vi "Main.vi"(8 "MaxPulse_Path":path, 9 "SingleMeasurement_Path":path, 10 "Optometer cfg file":path=path "C:/Gigahertz-Optik/config/TR9600MPEconfig.gdf", 11 "deviceName":string="TR9600_57976") -> (0 "Pulse End (ms)":dbl format="%.4f", 1 "Pulse Begin (ms)":dbl format="%.4f", 2 "Pulse_Time (µs)":dbl format="%.2f", 3 "Pulse_Energy (V/s)":dbl)   [LabVIEW 2018]
uses:
  <userlib>/Gigahertz-Optik/GOMDTR9600/GOMDTR9600.lvlib
panel:
  out "Progress":i32
  out "Single Measurement":cluster{dbl[], dbl[]}(graph) caption="Spectrum"
  out "State":i32
  in  "Resolution":u32=10000000
  out "Maximum Pulse":cluster{i32[], dbl[]}(graph) caption="Spectrum"
  out "Status":string
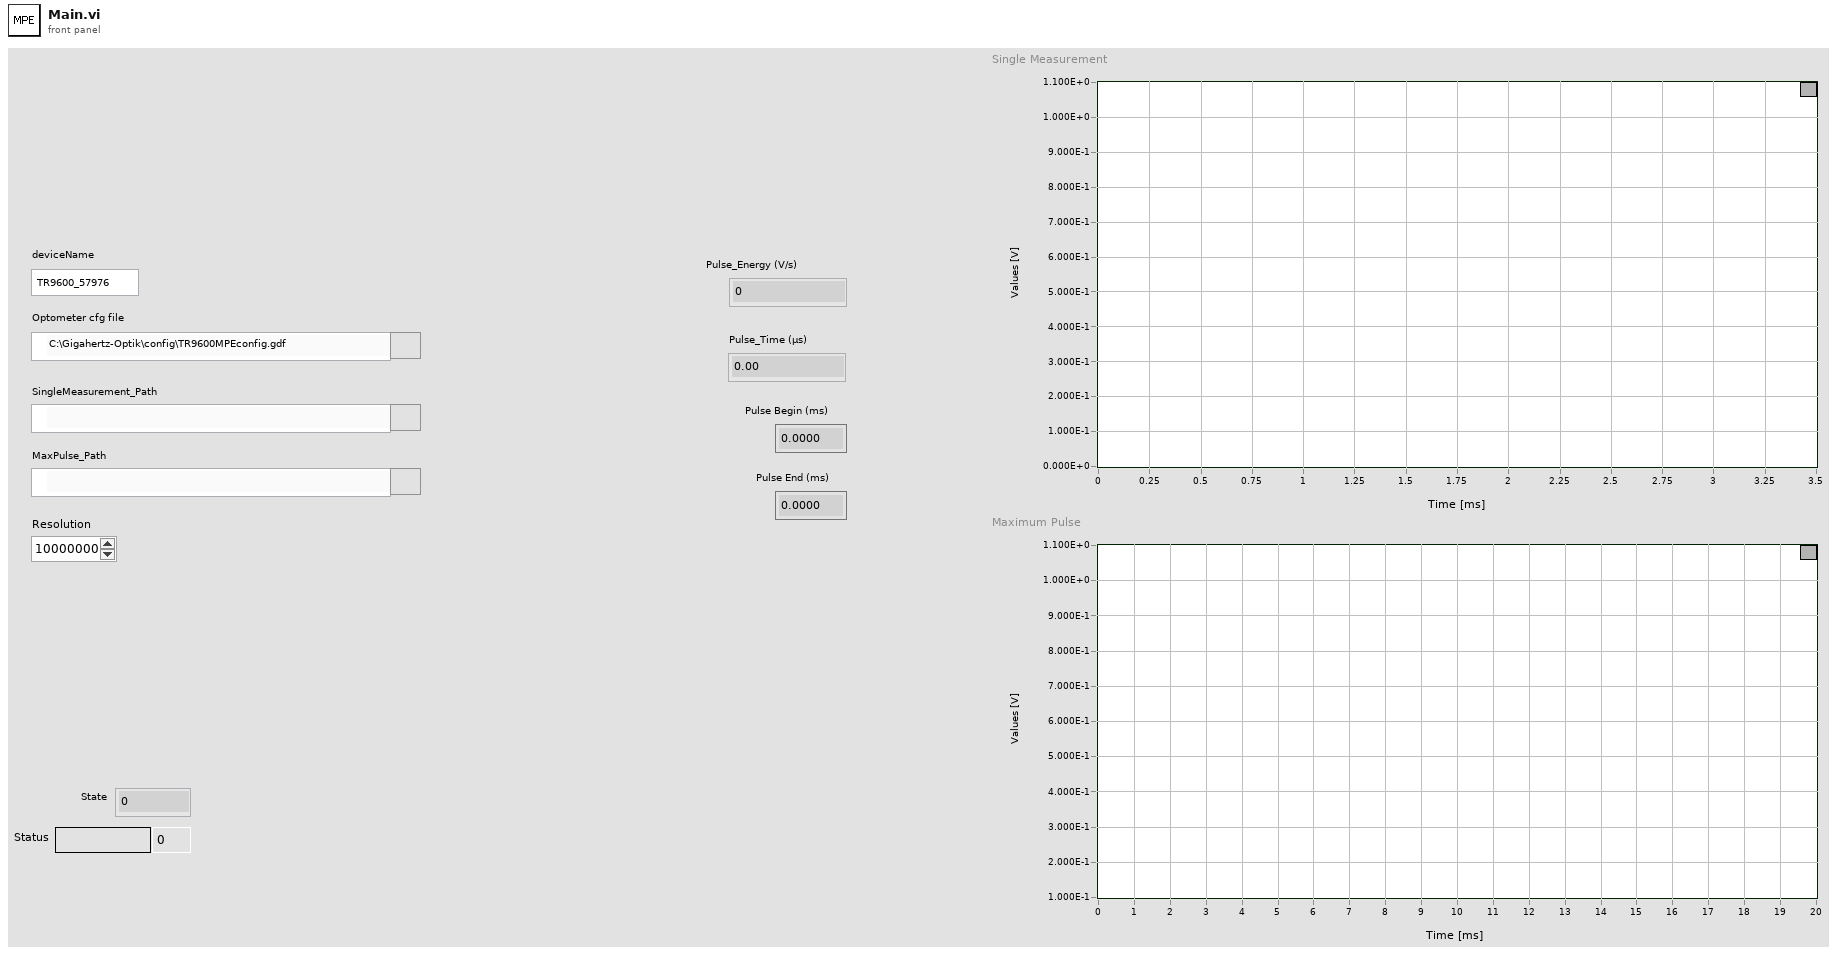
[diagram p1: front panel]
types:
  T1 = cluster{"address":i32, "mean value":dbl, "min value":dbl, "max value":dbl}[][]
  T2 = typedef "imagedata.ctl" = cluster{"image type":i32, "image depth":i32, "image":u8[], "mask":u8[], "colors":u32[], "Rectangle":cluster{"left":i16, "top":i16, "right":i16, "bottom":i16}}
  T3 = enum32{"invalid app kind", "Development System", "Run Time System", "Student Edition", "Embedded LabVIEW", "Evaluation", "Custom"}
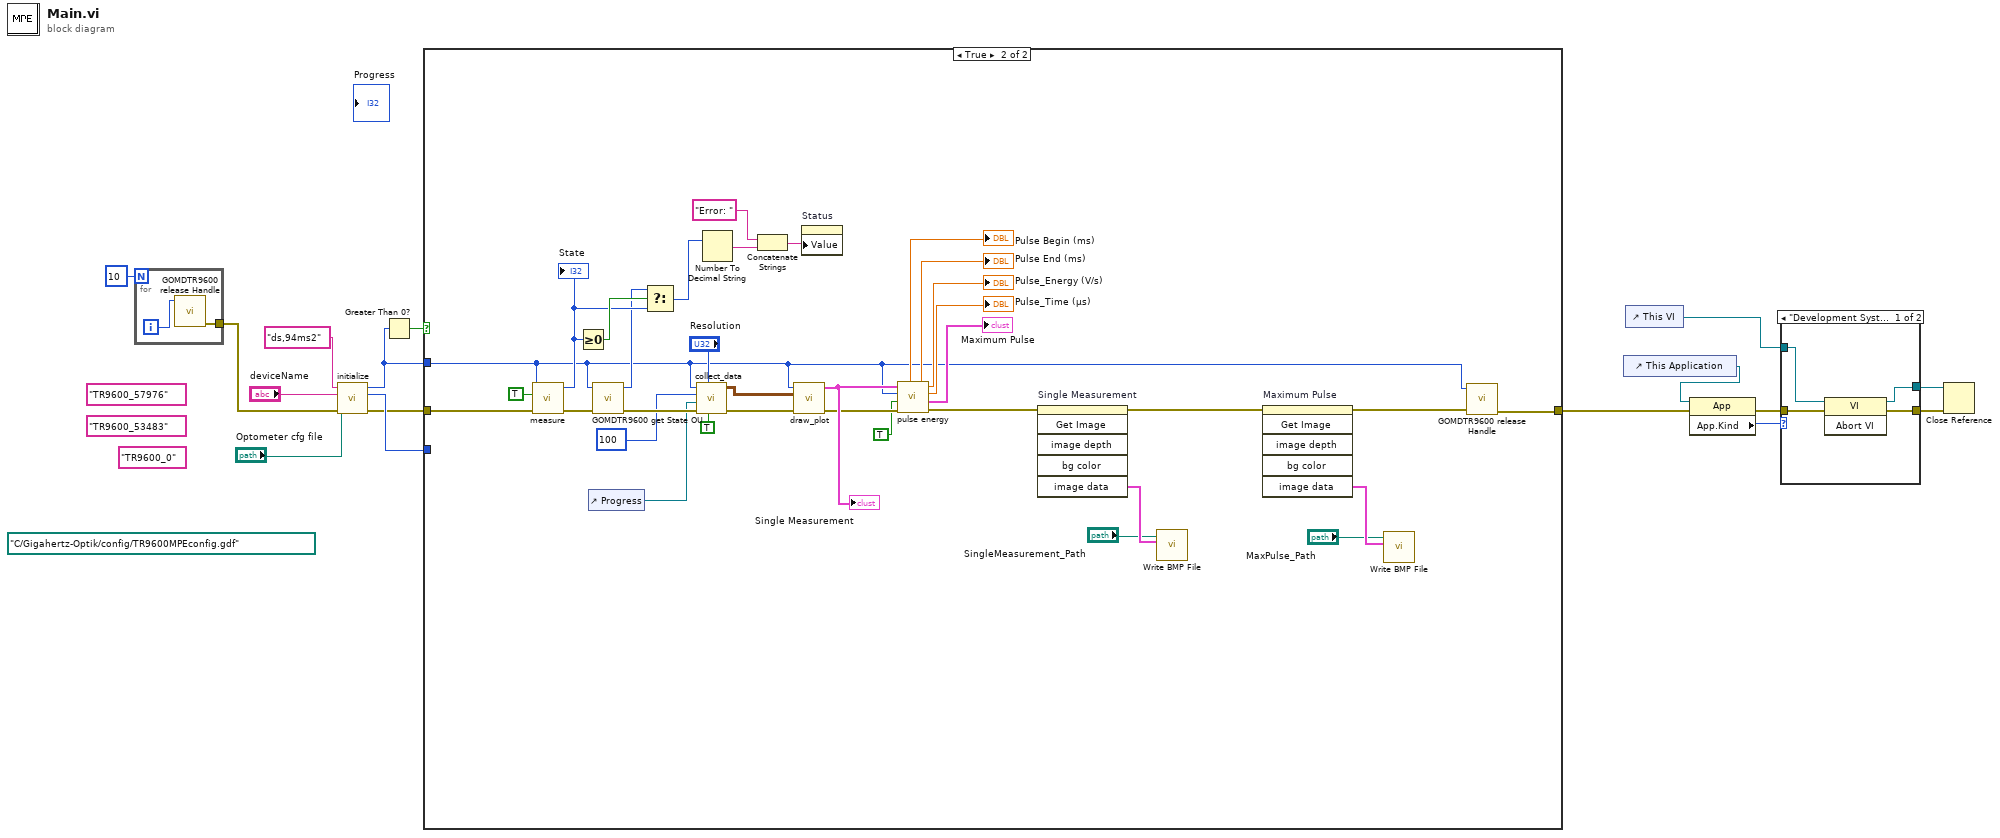
[diagram p0: block diagram]
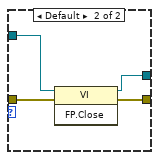
[diagram p2: hidden frame]
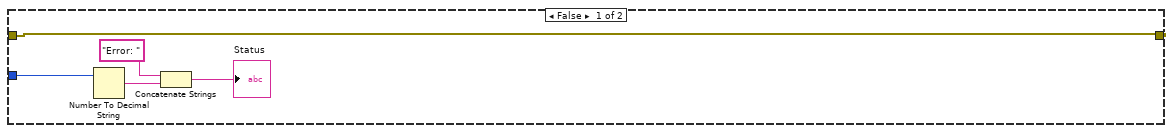
[diagram p3: hidden frame]
diagram:
  (unwired) "TR9600_53483" ("deviceName")
  (unwired) "TR9600_57976" ("deviceName")
  (unwired) path "C:/Gigahertz-Optik/config/TR9600MPEconfig.gdf" ("filename")
  (unwired) "TR9600_0" ("deviceName")
  n1 = for {
    N: 10 -> [_]
    tunnel: [w17] -> w4
    i -> [w18]
    n2 = call <userlib>:"GOMDTR9600 release Handle.vi"("handle"=w18) -> ("error out"=w17:errorcluster)  [unwired: 9 in, 1 out]
  }
  n3 = call "initialize.vi"("error in (no error)"=w4, "Optometer cfg file"="Optometer cfg file", "deviceName"="deviceName", "password"="ds,94ms2") -> ("error out"=w6:errorcluster, "function return"=w7:i32, "handle"=w3:i32)  [unwired: 5 in]
  n4 = Greater Than 0?(x=w3) -> (x > 0?=w16:bool)
  n5 = case shown="True" w16 {
    tunnel: w3 -> [_ w31]
    tunnel: w6 -> [w19 w57]
    tunnel: w7 -> [w23 _]
    tunnel: [w19 w32] -> w10
    frame False {
      n6 = Number To Decimal String(number=w23) -> (decimal integer string=w21:string)  [unwired: 1 in]
      n7 = Concatenate Strings("Error: ", w21) -> (→"Status":string)
    }
    frame True {
      n8 = call "measure.vi"("error in (no error)"=w57, "Measure"=TRUE, "handle"=w31) -> ("error out"=w52:errorcluster, "state"=w49:i32)  [unwired: 7 in]
      "State" <- w49
      n9 = Greater Or Equal To 0?(x=w49) -> (x >= 0?=w50:bool)
      n10 = control-ref of="Progress"() -> (w46:refnum<vi>)
      n11 = call <userlib>:"GOMDTR9600 get State OU.vi"("error in (no error)"=w52, "handle"=w31) -> ("error out"=w51:errorcluster, "value"=w48:i32)  [unwired: 7 in, 1 out]
      n12 = Select(t=w48, s=w50, f=w49) -> (s? t:f=w47:i32)
      n13 = call "collect_data.vi"("data?"=TRUE, "Resolution"="Resolution", "error in (no error)"=w51, "progress"=w46, "No. of values"=100, "handle"=w31) -> ("error out"=w56:errorcluster, "Dataset"=w42:T1)  [unwired: 4 in]
      n14 = Number To Decimal String(number=w47) -> (decimal integer string=w53:string)  [unwired: 1 in]
      n15 = Concatenate Strings("Error: ", w53) -> (w55:string)
      n16 = call "draw_plot.vi"("error in (no error)"=w56, "Dataset"=w42, "handle"=w31) -> ("error out"=w37:errorcluster, "Plot"=w38:cluster{dbl[], dbl[]})  [unwired: 7 in]
      "Single Measurement" <- w38
      n17 = property on="Status" class="Str"("Value"=w55) -> ()  [unwired: 2 in, 2 out]
      n18 = call "pulse energy.vi"("error in (no error)"=w37, "Boolean"=TRUE, "handle"=w31, "Spectrum"=w38) -> ("error out"=w26:errorcluster, "MaxPulse"=→"Maximum Pulse":cluster{i32[], dbl[]}, "Pulse_time"=→"Pulse_Time (µs)":dbl, "PulseEnergy"=→"Pulse_Energy (V/s)":dbl, "Pulse End"=→"Pulse End (ms)":dbl, "Pulse Begin"=→"Pulse Begin (ms)":dbl)  [unwired: 2 in]
      n19 = invoke on="Single Measurement" class="XYGraph (strict)" method="Get Image"(error in=w26) -> (error out=w25:errorcluster, "image data"=w30:T2)  [unwired: 5 in, 4 out]
      n20 = call <vilib>:"Write BMP File.vi"("image data"=w30, "path to BMP file"="SingleMeasurement_Path") -> ()  [unwired: 8 in, 2 out]
      n21 = invoke on="Maximum Pulse" class="XYGraph (strict)" method="Get Image"(error in=w25) -> (error out=w24:errorcluster, "image data"=w28:T2)  [unwired: 5 in, 4 out]
      n22 = call <vilib>:"Write BMP File.vi"("image data"=w28, "path to BMP file"="MaxPulse_Path") -> ()  [unwired: 8 in, 2 out]
      n23 = call <userlib>:"GOMDTR9600 release Handle.vi"("error in (no error)"=w24, "handle"=w31) -> ("error out"=w32:errorcluster)  [unwired: 8 in, 1 out]
    }
  }
  n24 = control-ref of="This Application"() -> (w9:refnum<vi>)
  n25 = control-ref of="This VI"() -> (w11:refnum<vi>)
  n26 = property class="App"(reference=w9, error in=w10) -> (error out=w14:errorcluster, "App.Kind"=w15:T3)  [unwired: 1 out]
  n27 = case shown="\"Development System\"" w15 {
    tunnel: w14 -> [w61 w65]
    tunnel: [w59 w63] -> w12
    tunnel: w11 -> [w58 w64]
    tunnel: [w60 w62] -> w13
    frame "Development System" {
      n28 = invoke class="VI" method="Abort VI"(reference=w58, error in=w61) -> (reference out=w60:refnum<vi>, error out=w59:errorcluster)  [unwired: 1 in, 1 out]
    }
    frame Default {
      n29 = invoke class="VI" method="FP.Close"(reference=w64, error in=w65) -> (reference out=w62:refnum<vi>, error out=w63:errorcluster)  [unwired: 1 in, 1 out]
    }
  }
  n30 = Close Reference(reference=w13, error in (no error)=w12) -> ()  [unwired: 1 out]
